vi "指定范围的随机数(dbl).vi"(6 "下限 (0.00)":dbl format="%.2f", 7 "上限 (1.00)":dbl=1.0 format="%.2f", 8 "Error In":errorcluster caption="错误输入") -> (0 "Error Out":errorcluster caption="错误输出", 3 "随机数":dbl format="%.2f")   [LabVIEW 2013]
doc: "功能：\n\n产生指定范围的<b>随机数</b>。\n\n\n\n\n\ncsxcs_366创建"
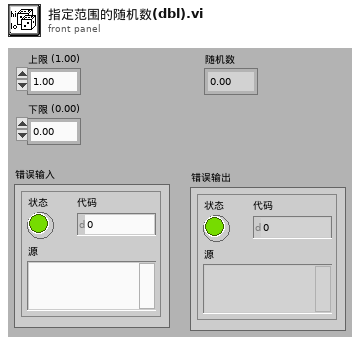
[diagram p1: front panel]
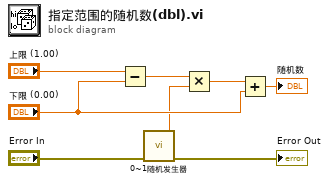
[diagram p0: block diagram]
diagram:
  n1 = Subtract(x="上限 (1.00)", y="下限 (0.00)") -> (x-y=w6:dbl)
  n2 = call-poly "0~1随机发生器.vi"("Error In"="Error In") -> ("Error Out"=→"Error Out":errorcluster, "Rand(0-1)"=w3:dbl)  [unwired: 9 in]
  n3 = Multiply(x=w6, y=w3) -> (x*y=w4:dbl)
  n4 = Add(x=w4, y="下限 (0.00)") -> (x+y=→"随机数":dbl)
